vi "Attemp driver connection.vi"(8 "error in (no error)":errorcluster, 11 "COM port in":refnum<visa-resource-name>) -> (0 "error out":errorcluster, 3 "COM port out":refnum<visa-resource-name>)   [LabVIEW 2020]
doc: "Attempts a connection to a MT694B piezo driver. Returns error 5003 if the device at the specified port is not the intended driver."
uses:
  <vilib>/Utility/error.llb/Error Cluster From Error Code.vi
  <vilib>/Instr/_visa.llb/VISA Configure Serial Port (Instr).vi
  <vilib>/ErrorRing/Error Ring.xnode
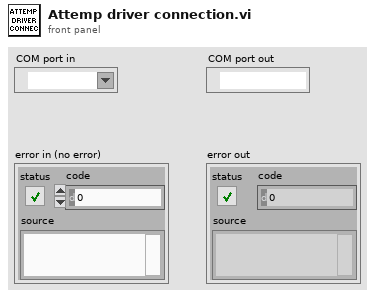
[diagram p1: front panel]
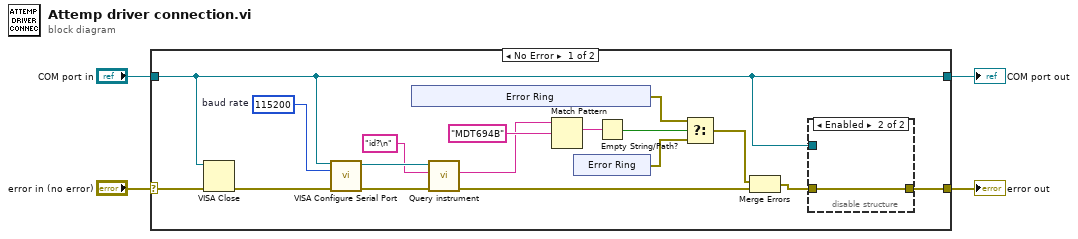
[diagram p0: block diagram]
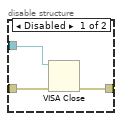
[diagram p2: hidden frame]
diagram:
  n1 = case shown="No Error" "error in (no error)" {
    selector: "error in (no error)" -> [w20 w33]
    tunnel: "COM port in" -> [w5 w32]
    tunnel: [w11 w33] -> w3
    tunnel: [w5 w32] -> w1
    frame No Error {
      w19 = u32 115200  # baud rate
      n2 = VISA Close(VISA resource name=w5, error in (no error)=w20) -> (error out=w21:errorcluster)
      n3 = call-poly "VISA Configure Serial Port"("VISA resource name"=w5, "baud rate (9600)"=w19, "error in (no error)"=w21) -> ("VISA resource name out"=w9:refnum<visa-resource-name>, "error out"=w10:errorcluster)  [unwired: 11 in]
      n4 = xnode "Error Ring"() -> ("error out"=w14:errorcluster)
      n5 = call "Query instrument.vi"("error in (no error)"=w10, "Command"="id?\n" ("write buffer"), "VISA Refnum in"=w9) -> ("error out"=w7:errorcluster, "read buffer"=w6:string)  [unwired: 6 in, 1 out]
      n6 = Match Pattern(string=w6, regular expression="MDT694B") -> (match substring=w17:string)  [unwired: 1 in, 3 out]
      n7 = xnode "Error Ring"() -> ("error out"=w15:errorcluster)
      n8 = Empty String/Path?(string/path=w17) -> (empty?=w16:bool)
      n9 = Select(t=w14, s=w16, f=w15) -> (s? t:f=w13:errorcluster)
      n10 = Merge Errors(w13, w7) -> (w12:errorcluster)
      n11 = disable-structure shown="Enabled" {
        disable-tunnel: w12 -> [w30 w31]
        disable-tunnel: [w29 w31] -> w11
        disable-tunnel: w5 -> [w28 _]
        frame Disabled {
          n12 = VISA Close(VISA resource name=w28, error in (no error)=w30) -> (error out=w29:errorcluster)
        }
        frame Enabled {
        }
      }
    }
    frame Error {
    }
  }
  "error out" <- w3
  "COM port out" <- w1
